vi "Sensor Change Detection.vi"(6 "Start Value":dbl, 8 "Reset":bool, 11 "Input":bool) -> (3 "Output":dbl)   [LabVIEW 2015]
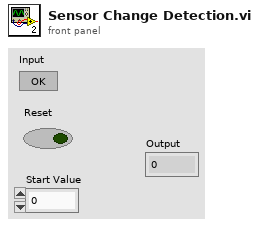
[diagram p1: front panel]
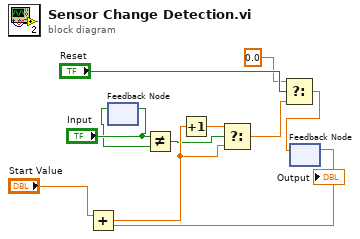
[diagram p0: block diagram]
diagram:
  n1 = feedback-in #1("Input") -> ()
  n2 = feedback #1() -> (w3:bool)  [unwired: 1 in]
  n3 = Not Equal?(x="Input", y=w3) -> (x != y?=w2:bool)
  n4 = feedback #2() -> (w5:dbl)  [unwired: 1 in]
  "Output" <- w5
  n5 = Add(x="Start Value", y=w5) -> (x+y=w7:dbl)
  n6 = Increment(x=w7) -> (x+1=w9:dbl)
  n7 = Select(t=w9, s=w2, f=w7) -> (s? t:f=w10:dbl)
  n8 = Select(t=0.0, s="Reset", f=w10) -> (s? t:f=w6:dbl)
  n9 = feedback-in #2(w6) -> ()
